vi "R_CARGACONDENSADOR_DAQ6008._2021vi.vi"() -> ()   [LabVIEW 2020]
uses:
  <vilib>/DAQmx/write.llb/DAQmx Write (Digital Bool 1Line 1Point).vi
  <vilib>/DAQmx/read.llb/DAQmx Read (Analog Wfm 1Chan NSamp).vi
  <vilib>/DAQmx/create/channels.llb/DAQmx Create Channel (AI-Voltage-Basic).vi
  <vilib>/DAQmx/configure/timing.llb/DAQmx Timing (Sample Clock).vi
  <vilib>/DAQmx/create/channels.llb/DAQmx Create Channel (DO-Digital Output).vi
  <vilib>/DAQmx/miscellaneous.llb/DAQmx Fill In Error Info.vi
  <resource>/objmgr/daqmx.rc
panel:
  out "task out":refnum<k21>
  in  "STOP":bool
  in  "Tab Control":T1(tab)
  out "Muestras":dbl(knob) scale=0.0..11000.0
  out "Tiempo":dbl(slide) caption="Elapsed Time (s)" scale=0.0..10.0
  in  "START":bool
  out "Boolean":bool
  out "Waveform Graph":dbl[](graph)
  in  "WRITE":bool caption="WRITE_CAPTION"
  in  "Resistencia":dbl format="%#_3g W"
  in  "Capacidad":ext format="%#_3g uF"
  in  "Vi":dbl format="%#_3g V"
  in  "Vf":dbl format="%#_3g V"
  out "FORMULA":cluster{"Boolean":bool}
  in  "t teórico":dbl(slide) scale=0.0..10.0
  out "Vins exp":dbl format="%#.3f V"
  out "t exp":dbl format="%#_3g s"
  in  "Vins teórica":dbl(slide) scale=0.0..5.0
  # "ADQUISICIÓN DE DATOS CON DAQ6008: CARGA DE CONDENSADOR"
  # "C(2021)"
  # "ANDRÉS R. PHILIPPS BENÍTEZ"
  # "PROYECTO CARGA CONDENSADOR MEDIANTE DAQ"
  # "- ESTE PROYECTO CONSISTE EN RECOGER DATOS MEDIANTE EL DAQ PROPIO DE LABVIEW. \n    - EL DATO A RECOGER SERÁ LA CARGA COMPLETA DE UN CONDENSADOR."
  # "OBJETIVO"
  # "MANUAL DE USO"
  # "GRÁFICA Y CALCULADORA\n\nEN ESTA PESTAÑA PODEMOS VISUALIZAR LA CARGA COMPLETA DEL CONDENSADOR Y REALIZAR EL CÁLCULO TEÓRICO DEL MISMO EN EL ORDEN QUE SE DESEE.\n\nPARA ESTIMAR EL VALOR TEORICO EN EL INSTANTE DE LA CARGA QUE DESEEMOS, SON NECESARIO LOS PARÁMETROS R, C, Vinicial y Vfinal DEL CONDENSADOR.\n\nPARA VISUALIZAR LA GRÁFICA, ES NECESARIO PULSAR EL BOTÓN 'START'. AL PULSARLO, SE ACTIVARÁ EL RELÉ QUE DA PASO A LA CARGA DEL CONDENSADOR. DE FORMA SIMULTÁNEA, SE IRÁ  ADQUIRIENDO MUESTRAS DE TENSIÓN DURANTE 10 SEGUNDOS.\nPOSTERIORMENTE, SERÁ PLASMADO EN LA GRÁFICA."
  # "ESQUEMA ELÉCTRICO\n\nEN ESTA PESTAÑA PODEMOS\n VER LOS ESQUEMAS \nELÉCTRICOS DE LA CARGA \nY DESCARGA DEL \nCONDENSADOR."
  # "ESQUEMA ELECTRICO REALIZADO EN PROTEUS"
  # "CONDENSADOR DESCARGADO"
  # "CONDENSADOR CARGADO"
  # "TIEMPO"
  # "Vins calculado"
  # "Vins"
  # "Nº DE MUESTRAS"
  # "TIEMPO"
  # "TIEMPO MUESTREO"
  # "R"
  # "Vi"
  # "C"
  # "Vf"
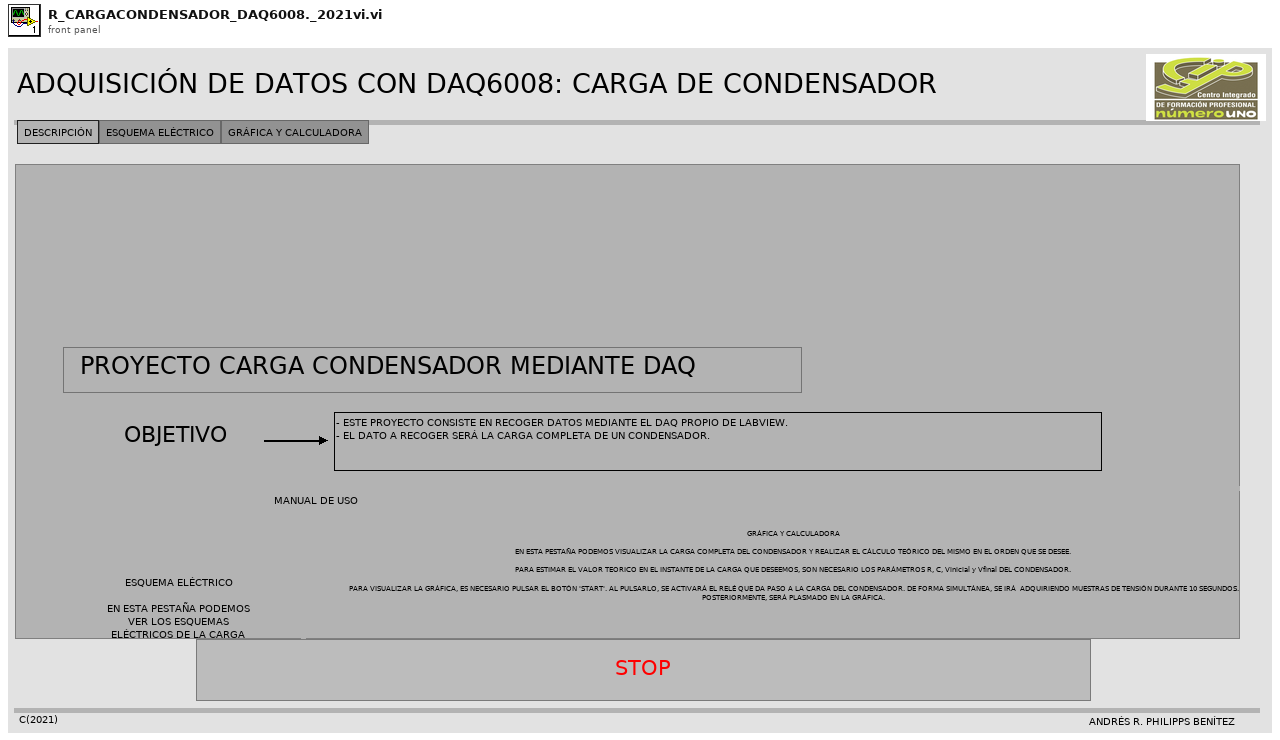
[diagram p1: front panel]
types:
  T1 = enum32{"DESCRIPCIÓN", "ESQUEMA ELÉCTRICO", "GRÁFICA Y CALCULADORA"}
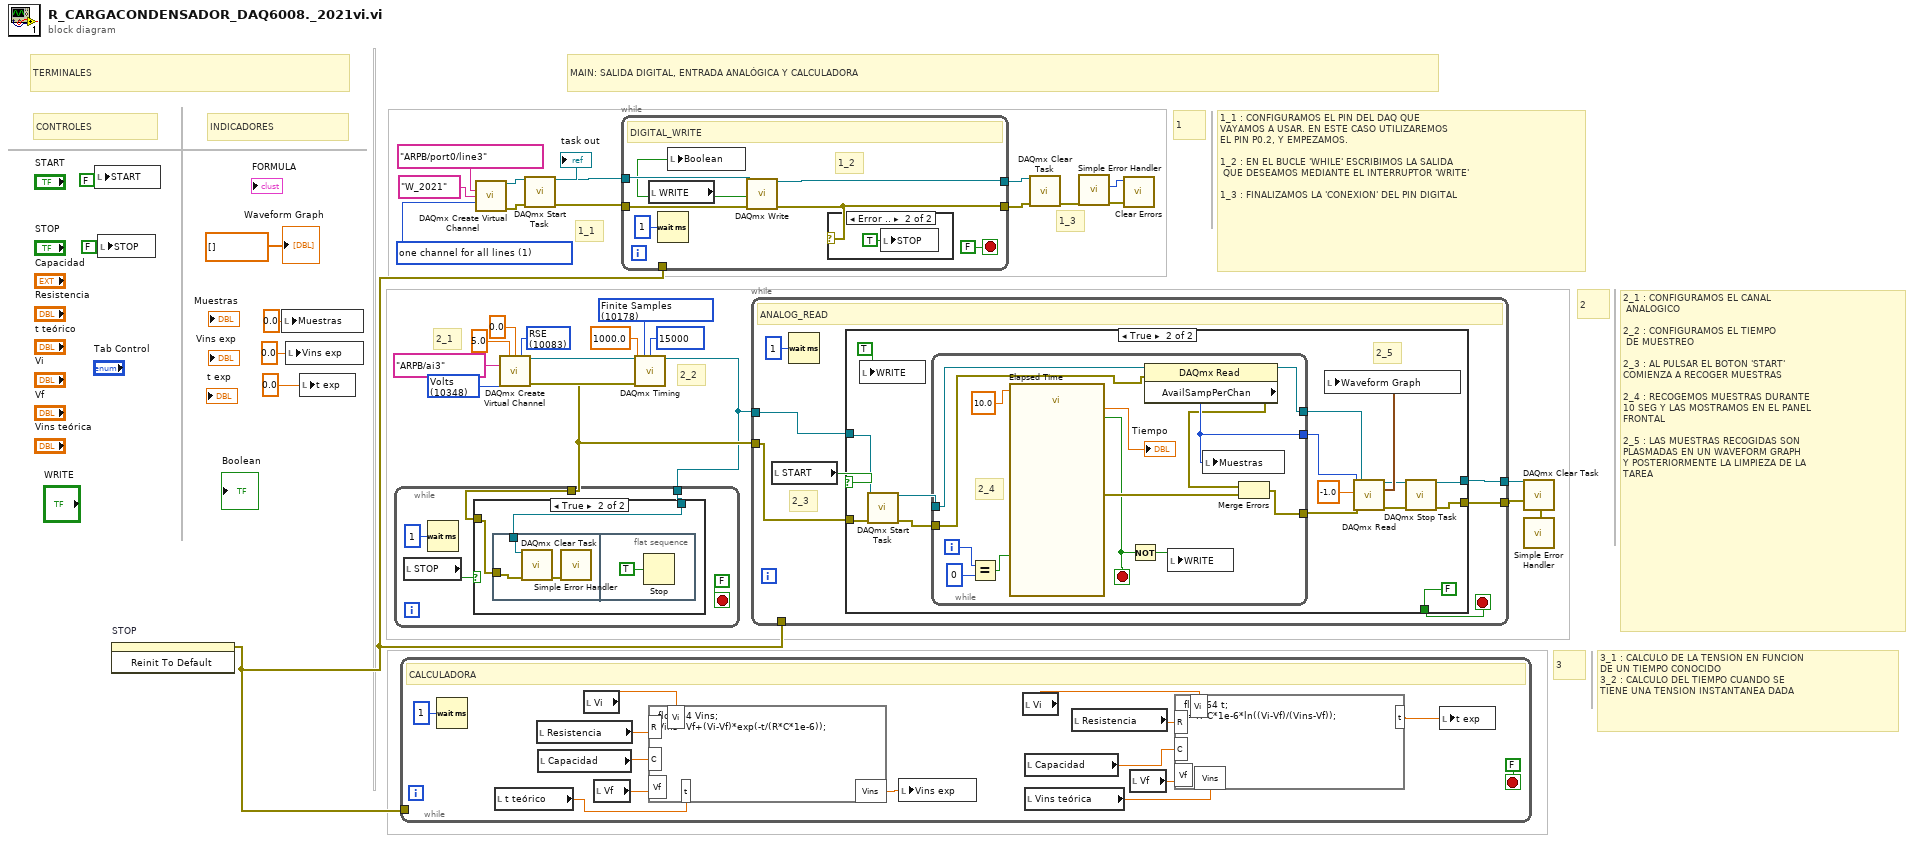
[diagram p0: block diagram]
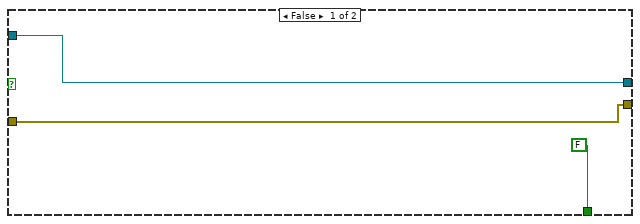
[diagram p4: hidden frame]
diagram:
  w14 = 1 items=["one channel for each line", "one channel for all lines"] ("line grouping")
  w28 = 10178 items=["Finite Samples"=10178, "Continuous Samples"=10123, "Hardware Timed Single Point"=12522] ("sample mode")
  w33 = 10348 items=["Volts"=10348, "From Custom Scale"=10065] ("units")
  w32 = 10083 items=["Default"=-1, "RSE"=10083, "Differential"=10106, "Pseudodifferential"=12529] ("output terminal configuration")
  # "MAIN: SALIDA DIGITAL, ENTRADA ANALÓGICA Y CALCULADORA"
  # "3_1 : CALCULO DE LA TENSION EN FUNCION\nDE UN TIEMPO CONOCIDO\n3_2 : CALCULO DEL TIEMPO CUANDO SE \nTIENE UNA TENSION INSTANTANEA DADA"
  # "3"
  # "2_2"
  # "2_1 : CONFIGURAMOS EL CANAL\n ANALOGICO\n\n2_2 : CONFIGURAMOS EL TIEMPO\n DE MUESTREO\n\n2_3 : AL PULSAR EL BOTON 'START' \nCOMIENZA A RECOGER MUESTRAS\n\n2_4 : RECOGEMOS MUESTRAS DURANTE \n10 SEG Y LAS MOSTRAMOS EN EL PANEL \nFRONTAL\n\n2_5 : LAS MUESTRAS RECOGIDAS SON \nPLASMADAS EN UN WAVEFORM GRAPH\nY POSTERIORMENTE LA LIMPIEZA DE LA \nTAREA"
  # "2_1"
  # "2"
  # "1_1 : CONFIGURAMOS EL PIN DEL DAQ QUE \nVAYAMOS A USAR. EN ESTE CASO UTILIZAREMOS \nEL PIN P0.2, Y EMPEZAMOS.\n\n1_2 : EN EL BUCLE 'WHILE' ESCRIBIMOS LA SALIDA\n QUE DESEAMOS MEDIANTE EL INTERRUPTOR 'WRITE'\n\n1_3 : FINALIZAMOS LA 'CONEXION' DEL PIN DIGITAL"
  # "1_3"
  # "1_1"
  # "1"
  # "INDICADORES"
  # "CONTROLES"
  # "TERMINALES"
  n1 = local write "START"(FALSE ("START")) -> ()
  n2 = local write "STOP"(FALSE ("STOP")) -> ()
  n3 = invoke on="STOP" class="Bool (strict)" method="Reinit To Default"() -> (error out=w1:errorcluster)  [unwired: 3 in, 2 out]
  n4 = local write "Muestras"(0.0 ("Muestras")) -> ()
  n5 = local write "Vins exp"(0.0 ("Vins")) -> ()
  n6 = local write "t exp"(0.0 ("Tiempo de carga")) -> ()
  n7 = while {
    tunnel: w1 -> [_]
    stop <- FALSE stop-if-true
    # "3_2"
    # "3_1"
    # "CALCULADORA"
    n8 = Wait (ms)(milliseconds to wait=u32 1) -> ()  [unwired: 1 out]
    n9 = local read "t teórico"() -> (w41:dbl)
    n10 = local read "Resistencia"() -> (w44:dbl)
    n11 = local read "Capacidad"() -> (w45:ext)
    n12 = local read "Vi"() -> (w43:dbl)
    n13 = local read "Vf"() -> (w42:dbl)
    n14 = formula code="float64 Vins;\nVins=Vf+(Vi-Vf)*exp(-t/(R*C*1e-6));"("Vi"=w43, "R"=w44, "C"=w45, "Vf"=w42, "t"=w41) -> ("Vins"=w46:dbl)
    n15 = local write "Vins exp"(w46) -> ()
    n16 = local read "Vi"() -> (w39:dbl)
    n17 = local read "Capacidad"() -> (w37:ext)
    n18 = local read "Vins teórica"() -> (w35:dbl)
    n19 = local read "Resistencia"() -> (w38:dbl)
    n20 = local read "Vf"() -> (w36:dbl)
    n21 = formula code="float64 t;\nt=R*C*1e-6*ln((Vi-Vf)/(Vins-Vf));"("Vi"=w39, "R"=w38, "C"=w37, "Vf"=w36, "Vins"=w35) -> ("t"=w40:dbl)
    n22 = local write "t exp"(w40) -> ()
  }
  n23 = call-poly <vilib>:"DAQmx Create Virtual Channel.vi"("lines"=tag "ARPB/port0/line3", "name to assign"="W_2021", "line grouping"=w14) -> ("task out"=w13:refnum<k21>, "error out"=w12:errorcluster)  [unwired: 11 in]
  "task out" <- w13
  n24 = call-poly <vilib>:"DAQmx Create Virtual Channel.vi"("maximum value"=5.0, "minimum value"=0.0, "input terminal configuration"=w32, "physical channels"=tag "ARPB/ai3", "units"=w33) -> ("task out"=w23:refnum<k21>, "error out"=w24:errorcluster)  [unwired: 9 in]
  n25 = call <vilib>:"DAQmx Start Task.vi"("task/channels in"=w13, "error in"=w12) -> ("task out"=w11:refnum<k21>, "error out"=w10:errorcluster)  [unwired: 12 in]
  n26 = while {
    tunnel: w11 -> [w54]
    tunnel: w10 -> [w53]
    tunnel: [w52] -> w9
    tunnel: [w50] -> w8
    tunnel: w1 -> [_]
    stop <- FALSE stop-if-true
    # "1_2"
    # "DIGITAL_WRITE"
    n27 = local read "WRITE"() -> (w49:bool)
    n28 = Wait (ms)(milliseconds to wait=u32 1) -> ()  [unwired: 1 out]
    n29 = local write "Boolean"(w49) -> ()
    n30 = call-poly <vilib>:"DAQmx Write.vi"("task/channels in"=w54, "data"=w49, "error in"=w53) -> ("task out"=w52:refnum<k21>, "error out"=w50:errorcluster)  [unwired: 10 in, 1 out]
    n31 = case shown="Error .." w50 {
      frame No Error {
      }
      frame Error {
        n32 = local write "STOP"(TRUE ("stop")) -> ()
      }
    }
  }
  n33 = call-poly <vilib>:"DAQmx Timing.vi"("task/channels in"=w23, "sample mode"=w28, "samples per channel"=15000, "rate"=1000.0, "error in"=w24) -> ("task out"=w2:refnum<k21>, "error out"=w3:errorcluster)  [unwired: 9 in]
  n34 = while {
    tunnel: w3 -> [w60]
    tunnel: w2 -> [w59]
    stop <- FALSE stop-if-true
    n35 = local read "STOP"() -> (w58:bool)
    n36 = Wait (ms)(milliseconds to wait=u32 1) -> ()  [unwired: 1 out]
    n37 = case shown="True" w58 {
      tunnel: w60 -> [_ w63]
      tunnel: w59 -> [_ w62]
      frame False {
      }
      frame True {
        n38 = flat-sequence {
          tunnel: w63 -> [w65]
          tunnel: w62 -> [w66]
          frame #0 {
            n39 = call <vilib>:"DAQmx Clear Task.vi"("task in"=w66, "error in"=w65) -> ("error out"=w64:errorcluster)  [unwired: 13 in]
            n40 = call <vilib>:"Simple Error Handler.vi"("error in (no error)"=w64) -> ()  [unwired: 4 in, 5 out]
          }
          frame #1 {
            n41 = Stop(stop? (T)=TRUE) -> ()
          }
        }
      }
    }
  }
  n42 = while {
    tunnel: w2 -> [w71]
    tunnel: w3 -> [w72]
    tunnel: [w70] -> w18
    tunnel: [w68] -> w17
    tunnel: w1 -> [_]
    stop <- w69 stop-if-true
    # "2_3"
    # "ANALOG_READ"
    n43 = local read "START"() -> (w73:bool)
    n44 = Wait (ms)(milliseconds to wait=u32 1) -> ()  [unwired: 1 out]
    n45 = case shown="True" w73 {
      tunnel: w72 -> [w75 w83]
      tunnel: w71 -> [w77 w84]
      tunnel: [w77 w79] -> w70
      tunnel: [FALSE FALSE] -> w69
      tunnel: [w75 w78] -> w68
      frame False {
      }
      frame True {
        # "2_5"
        n46 = local write "WRITE"(TRUE ("WRITE 2")) -> ()
        n47 = call <vilib>:"DAQmx Start Task.vi"("task/channels in"=w84, "error in"=w83) -> ("task out"=w86:refnum<k21>, "error out"=w85:errorcluster)  [unwired: 12 in]
        n48 = while {
          tunnel: [w100] -> w91
          tunnel: [w96] -> w90
          tunnel: w86 -> [w105]
          tunnel: w85 -> [w99]
          tunnel: [w101] -> w88
          i -> [w103]
          stop <- w94 stop-if-true
          # "2_4"
          n49 = Equal?(x=w103, y=0) -> (x = y?=w104:bool)
          n50 = call "Elapsed Time"("Time Target (s)"=10.0, "Reset"=w104) -> ("Elapsed Time (s)"=→"Tiempo":dbl, "Time has Elapsed"=w94:bool, "error out"=w98:errorcluster)  [unwired: 10 in, 5 out]
          n51 = Not(x=w94) -> (.not. x?=w93:bool)
          n52 = property class="DAQmx Read"(reference=w105, error in=w99) -> (reference out=w100:refnum<k21>, error out=w97:errorcluster, "AvailSampPerChan"=w101:u32)
          n53 = local write "WRITE"(w93) -> ()
          n54 = local write "Muestras"(w101) -> ()
          n55 = Merge Errors(w97, w98) -> (w96:errorcluster)
        }
        n56 = call-poly <vilib>:"DAQmx Read.vi"("task/channels in"=w91, "number of samples per channel"=w88, "timeout"=-1.0, "error in"=w90) -> ("task out"=w81:refnum<k21>, "data"=w89:waveform(dbl), "error out"=w80:errorcluster)  [unwired: 9 in]
        n57 = local write "Waveform Graph"(w89) -> ()
        n58 = call <vilib>:"DAQmx Stop Task.vi"("task/channels in"=w81, "error in"=w80) -> ("task out"=w79:refnum<k21>, "error out"=w78:errorcluster)  [unwired: 12 in]
      }
    }
  }
  n59 = call <vilib>:"DAQmx Clear Task.vi"("task in"=w9, "error in"=w8) -> ("error out"=w7:errorcluster)  [unwired: 13 in]
  n60 = call <vilib>:"Simple Error Handler.vi"("error in (no error)"=w7) -> ("code out"=w5:i32, "error out"=w6:errorcluster)  [unwired: 4 in, 3 out]
  n61 = call <vilib>:"Clear Errors.vi"("error in (no error)"=w6, "specific error code to clear (0: all)"=w5) -> ()  [unwired: 4 in, 2 out]
  n62 = call <vilib>:"DAQmx Clear Task.vi"("task in"=w18, "error in"=w17) -> ("error out"=w19:errorcluster)  [unwired: 13 in]
  n63 = call <vilib>:"Simple Error Handler.vi"("error in (no error)"=w19) -> ()  [unwired: 4 in, 5 out]
  "Waveform Graph" <- dbl[] [] ("Waveform Graph")
